vi "Disabled&Enabled.vi"(8 "error in (no error)":errorcluster caption="错误输入（无错误）", 10 "Mode in":T1(ring), 11 "AllControls In":T2) -> (0 "error out":errorcluster caption="错误输出")   [LabVIEW 2017]
uses:
  Ctrls/AllControls.ctl
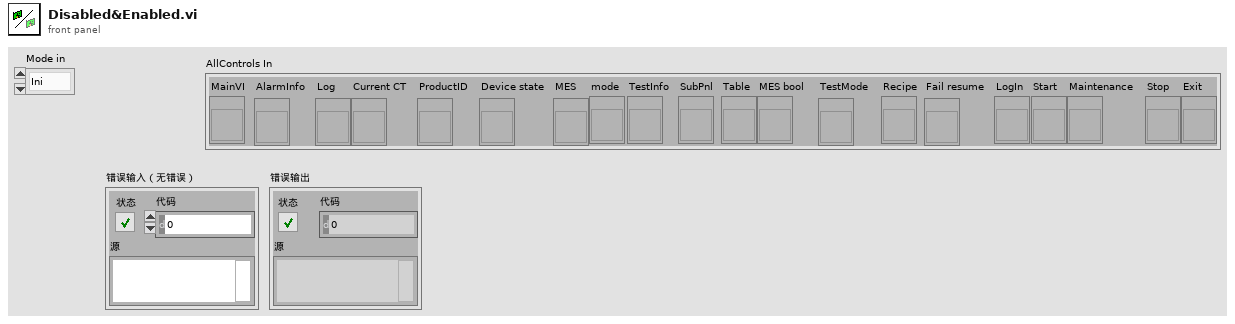
[diagram p1: front panel]
types:
  T1 = enum16{"Ini", "Standby", "Running", "Engineering"}
  T2 = typedef "AllControls.ctl" = cluster{"MainVI":refnum<vi>, "AlarmInfo":refnum<vi>, "Log":refnum<vi>, "Current CT":refnum<vi>, "ProductID":refnum<vi>, "Device state":refnum<vi>, "MES":refnum<vi>, "mode":refnum<vi>, "TestInfo":refnum<vi>, "SubPnl":refnum<vi>, "Table":refnum<vi>, "MES bool":refnum<vi>, "TestMode":refnum<vi>, "Recipe":refnum<vi>, "Fail resume":refnum<vi>, "LogIn":refnum<vi>, "Start":refnum<vi>, "Maintenance":refnum<vi>, "Stop":refnum<vi>, "Exit":refnum<vi>}
  T3 = enum8{"Enabled", "Disabled", "Disabled and Grayed Out"}
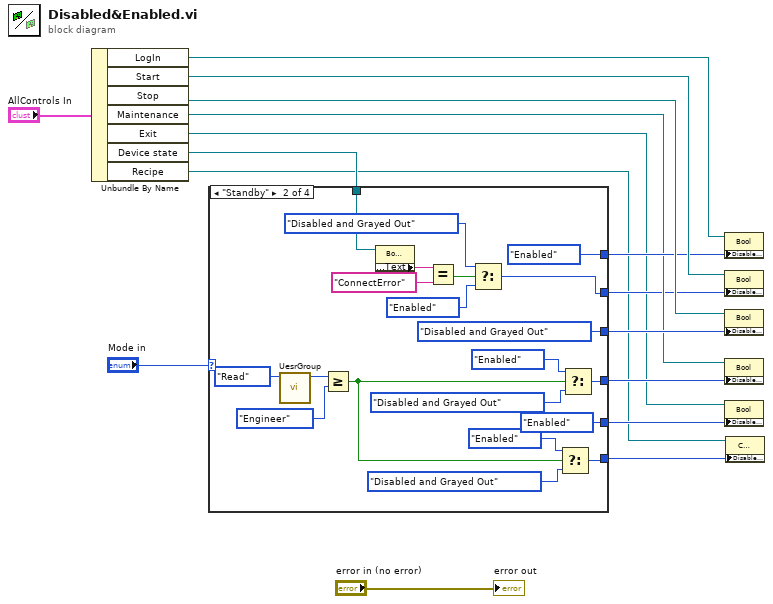
[diagram p0: block diagram]
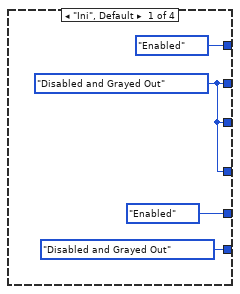
[diagram p2: hidden frame]
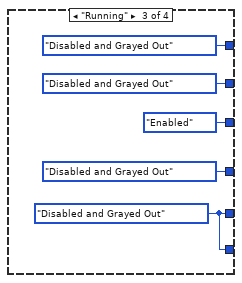
[diagram p3: hidden frame]
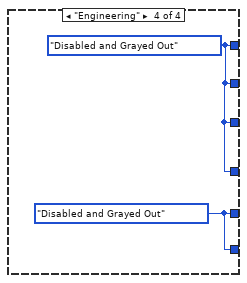
[diagram p4: hidden frame]
diagram:
  n1 = Unbundle By Name("AllControls In") -> ("LogIn"=w10:refnum<vi>, "Start"=w14:refnum<vi>, "Stop"=w13:refnum<vi>, "Maintenance"=w8:refnum<vi>, "Exit"=w4:refnum<vi>, "Device state"=w5:refnum<vi>, "Recipe"=w2:refnum<vi>)
  n2 = case shown="\"Standby\"" "Mode in" {
    tunnel: [w19 T3."Disabled and Grayed Out" ("禁用") T3."Enabled" ("禁用") w47] -> w12
    tunnel: [T3."Enabled" ("禁用") T3."Enabled" ("禁用") T3."Disabled and Grayed Out" ("禁用") w47] -> w11
    tunnel: [w19 w34 T3."Disabled and Grayed Out" ("禁用") w47] -> w9
    tunnel: [w19 w26 T3."Disabled and Grayed Out" ("禁用") w47] -> w7
    tunnel: w5 -> [_ w33 _ _]
    tunnel: [T3."Enabled" ("禁用") T3."Enabled" ("禁用") w41 w46] -> w3
    tunnel: [T3."Disabled and Grayed Out" ("禁用") w22 w41 w46] -> w1
    frame "Ini", Default {
      w19 = T3."Disabled and Grayed Out" ("禁用")
    }
    frame "Standby" {
      n3 = call "UesrGroup.vi"("Step"=enum16{"Initial", "Write", "Read"}."Read") -> ("User group out"=w40:enum16{"Operator", "Engineer", "Admin"})  [unwired: 9 in, 1 out]
      n4 = Greater Or Equal?(x=w40, y=enum16{"Operator", "Engineer", "Admin"}."Engineer" ("User group out")) -> (x >= y?=w21:bool)
      n5 = property class="Bool (严格)"(reference=w33) -> ("BoolText.Text"=w32:string)  [unwired: 1 in, 2 out]
      n6 = Equal?(x=w32, y="ConnectError") -> (x = y?=w30:bool)
      n7 = Select(t=T3."Disabled and Grayed Out" ("禁用"), s=w30, f=T3."Enabled" ("禁用")) -> (s? t:f=w26:T3)
      n8 = Select(t=T3."Enabled" ("禁用"), s=w21, f=T3."Disabled and Grayed Out" ("禁用")) -> (s? t:f=w22:T3)
      n9 = Select(t=T3."Enabled" ("禁用"), s=w21, f=T3."Disabled and Grayed Out" ("禁用")) -> (s? t:f=w34:T3)
    }
    frame "Running" {
      w41 = T3."Disabled and Grayed Out" ("禁用")
    }
    frame "Engineering" {
      w46 = T3."Disabled and Grayed Out" ("禁用")
      w47 = T3."Disabled and Grayed Out" ("禁用")
    }
  }
  n10 = property class="Bool"(reference=w10, "DisabledEnum"=w11) -> ()  [unwired: 1 in, 2 out]
  n11 = property class="Bool"(reference=w14, "DisabledEnum"=w7) -> ()  [unwired: 1 in, 2 out]
  n12 = property class="Bool"(reference=w13, "DisabledEnum"=w12) -> ()  [unwired: 1 in, 2 out]
  n13 = property class="Bool"(reference=w8, "DisabledEnum"=w9) -> ()  [unwired: 1 in, 2 out]
  n14 = property class="Bool"(reference=w4, "DisabledEnum"=w3) -> ()  [unwired: 1 in, 2 out]
  n15 = property class="CmbBox"(reference=w2, "DisabledEnum"=w1) -> ()  [unwired: 1 in, 2 out]
  "error out" <- "error in (no error)"
